vi "LED_Set_RGB.vi"(8 "B":dbl min=0.0 max=1.0 step=0.01 format="%#_13g", 9 "G":dbl min=0.0 max=1.0 step=0.01 format="%#_13g", 10 "R":dbl min=0.0 max=1.0 step=0.01 format="%#_13g", 11 "CANifierDevRef":T1) -> ()   [LabVIEW 2019]
uses:
  <vilib>/Rock Robotics/WPI/ThirdParty/Phoenix-LabVIEW/CANifier/CTRE_CANifier_LEDChannel.ctl
  <vilib>/Rock Robotics/WPI/ThirdParty/Phoenix-LabVIEW/CANifier/CTRE_CANifier_DeviceRef.ctl
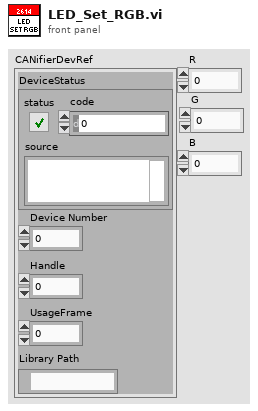
[diagram p1: front panel]
types:
  T1 = typedef "CTRE_CANifier_DeviceRef.ctl" = cluster{"DeviceStatus":errorcluster, "Device Number":u8, "Handle":u64, "UsageFrame":u32, "Library Path":path}
  T2 = typedef "CTRE_CANifier_LEDChannel.ctl" = enum32{"LEDChannelA", "LEDChannelB", "LEDChannelC"}
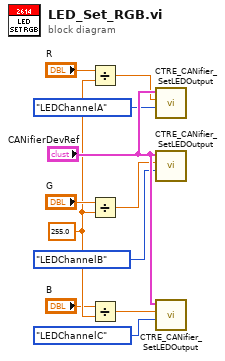
[diagram p0: block diagram]
diagram:
  w8 = 255.0 ("y")
  n1 = Divide(x="R", y=w8) -> (x/y=w3:dbl)
  n2 = Divide(x="G", y=w8) -> (x/y=w2:dbl)
  n3 = Divide(x="B", y=w8) -> (x/y=w1:dbl)
  n4 = call <vilib>:"CTRE_CANifier_SetLEDOutput.vi"("LEDChannel"=CTRE_CANifier_LEDChannel."LEDChannelA", "Percent Output"=w3, "CANifierDevRef"="CANifierDevRef") -> ()  [unwired: 7 in, 2 out]
  n5 = call <vilib>:"CTRE_CANifier_SetLEDOutput.vi"("LEDChannel"=CTRE_CANifier_LEDChannel."LEDChannelB", "Percent Output"=w2, "CANifierDevRef"="CANifierDevRef") -> ()  [unwired: 7 in, 2 out]
  n6 = call <vilib>:"CTRE_CANifier_SetLEDOutput.vi"("LEDChannel"=CTRE_CANifier_LEDChannel."LEDChannelC", "Percent Output"=w1, "CANifierDevRef"="CANifierDevRef") -> ()  [unwired: 7 in, 2 out]
